vi "LogUnhandledMessage.vi"(8 "error in (no error)":errorcluster, 9 "message":string, 10 "process":string, 11 "Qbus in":refnum<class "Qbus.lvclass">) -> (0 "error out":errorcluster)   [LabVIEW 2017, in "TraceLogger.lvlib"]
uses:
  <vilib>/addons/TraceLogger/TraceLogger.lvlib
  <vilib>/addons/Qbus/Qbus.lvclass
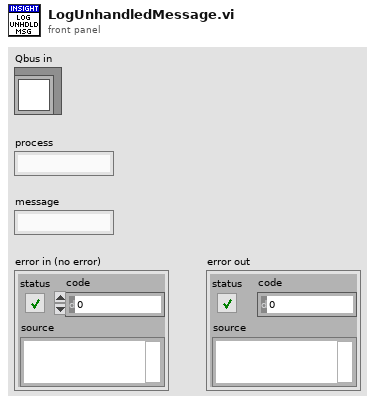
[diagram p1: front panel]
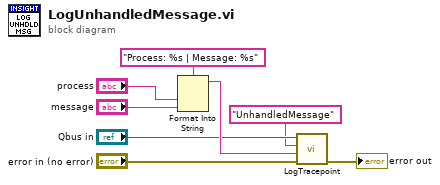
[diagram p0: block diagram]
diagram:
  n1 = Format Into String(format string="Process: %s | Message: %s", "process", "message") -> (resulting string=w8:string)  [unwired: 2 in, 1 out]
  n2 = call <vilib>:"LogTracepoint.vi"("error in (no error)"="error in (no error)", "log string"=w8, "tracepoint"="UnhandledMessage", "qbus in"="Qbus in") -> ("error out"=→"error out":errorcluster)  [unwired: 6 in, 1 out]
